vi "Set_TempHum_Calibration.vi"(2 "Path":path, 3 "Inside temp":dbl min=-7.0 max=7.0 step=0.01, 4 "Outside temp":dbl min=-7.0 max=7.0 step=0.01, 8 "Inside hum.":dbl, 9 "Outside hum":dbl) -> (0 "Cor. in temp":dbl, 1 "Cor. out temp":dbl, 5 "Cor. in hum":dbl, 6 "Cor. out hum":dbl, 7 "Calibration values set?":bool)   [LabVIEW 2012]
uses:
  <vilib>/Utility/config.llb/Write Key (Double).vi
  <vilib>/Utility/config.llb/Write Key (I32).vi
  VantagePro.dll
  <vilib>/Utility/config.llb/NI_LVConfig.lvlib
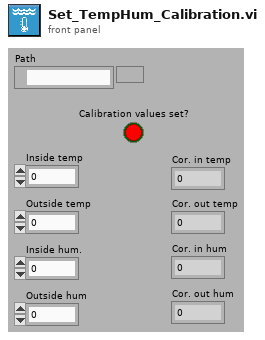
[diagram p1: front panel]
types:
  T1 = cluster{"In Temp":sgl, "Out Temp":sgl, "In Hum":u8, "Out Hum":u8, "Dum":i8, "Dum":i8, "Off In Temp":sgl, "Off Out Temp":sgl, "Off In Hum":i8, "Off Out Hum":i8}
  T2 = cluster{"In Temp":dbl, "Out Temp":dbl, "In Hum":dbl, "Out Hum":dbl}
  T3 = typedef "NI_LVConfig.lvlib/Config Data RefNum.ctl" = refnum<k1>
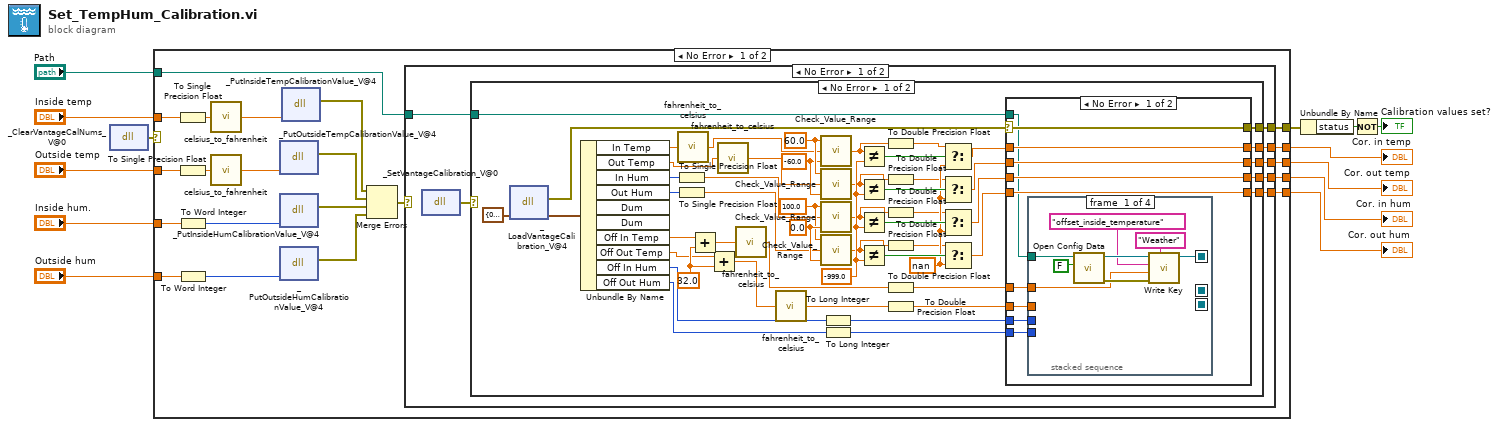
[diagram p0: block diagram]
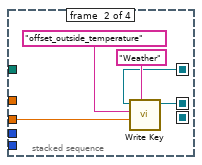
[diagram p2: hidden frame]
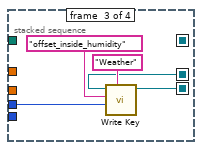
[diagram p3: hidden frame]
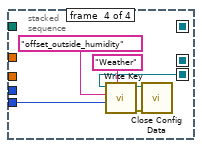
[diagram p4: hidden frame]
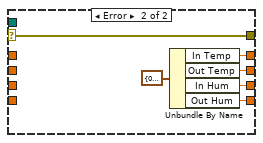
[diagram p5: hidden frame]
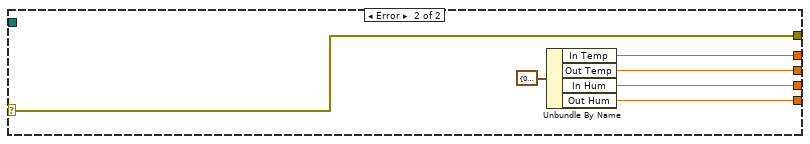
[diagram p6: hidden frame]
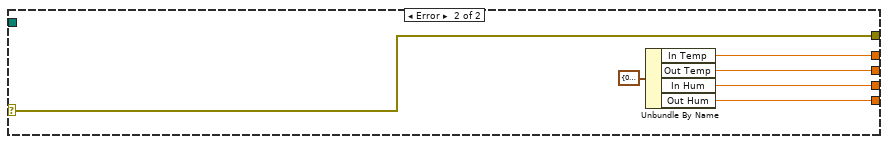
[diagram p7: hidden frame]
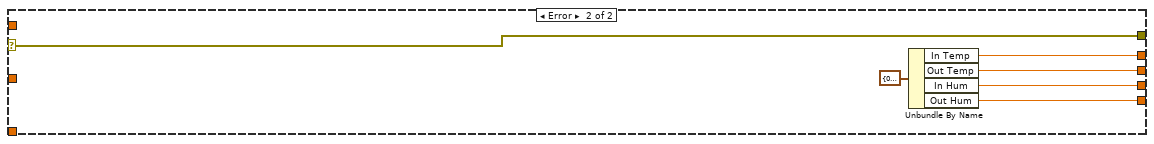
[diagram p8: hidden frame]
diagram:
  n1 = dll-call lib="C:/Users/Bob van Eijk/Desktop/LabView Projects 12/HiSPARC Weather Station/Develop/VantagePro.dll" fn="_ClearVantageCalNums_V@0" label="Clear Cal Nums"() -> (error out=w13:errorcluster)  [unwired: 4 in, 1 out]
  n2 = case shown="No Error" w13 {
    selector: w13 -> [_ w151]
    tunnel: "Inside temp" -> [w25 _]
    tunnel: "Inside hum." -> [w23 _]
    tunnel: "Outside temp" -> [w24 _]
    tunnel: "Outside hum" -> [w22 _]
    tunnel: "Path" -> [w31 _]
    tunnel: [w30 w151] -> w7
    tunnel: [w29 w149] -> w4
    tunnel: [w28 w148] -> w3
    tunnel: [w27 w147] -> w2
    tunnel: [w26 w146] -> w1
    frame No Error {
      n3 = To Single Precision Float(number=w25) -> (single precision float=w33:sgl)
      n4 = To Single Precision Float(number=w24) -> (single precision float=w34:sgl)
      n5 = To Word Integer(number=w23) -> (16bit integer=w15:i16)
      n6 = To Word Integer(number=w22) -> (16bit integer=w14:i16)
      n7 = call "celsius_to_fahrenheit.vi"("Celcius"=w33) -> ("Fahrenheit"=w21:sgl)
      n8 = call "celsius_to_fahrenheit.vi"("Celcius"=w34) -> ("Fahrenheit"=w16:sgl)
      n9 = dll-call lib="C:/Users/Bob van Eijk/Desktop/LabView Projects 12/HiSPARC Weather Station/Develop/VantagePro.dll" fn="_PutOutsideTempCalibrationValue_V@4" label="Put Out Temp Cal Val"("valValue"=w16) -> (error out=w19:errorcluster)  [unwired: 5 in, 1 out]
      n10 = dll-call lib="C:/Users/Bob van Eijk/Desktop/LabView Projects 12/HiSPARC Weather Station/Develop/VantagePro.dll" fn="_PutInsideHumCalibrationValue_V@4" label="Put In Hum Cal Val"("calValue"=w15) -> (error out=w18:errorcluster)  [unwired: 5 in, 1 out]
      n11 = dll-call lib="C:/Users/Bob van Eijk/Desktop/LabView Projects 12/HiSPARC Weather Station/Develop/VantagePro.dll" fn="_PutOutsideHumCalibrationValue_V@4" label="Put Out Hum Cal Val"("calValue"=w14) -> (error out=w17:errorcluster)  [unwired: 5 in, 1 out]
      n12 = dll-call lib="C:/Users/Bob van Eijk/Desktop/LabView Projects 12/HiSPARC Weather Station/Develop/VantagePro.dll" fn="_PutInsideTempCalibrationValue_V@4" label="Put In Temp Cal Val"("calValue"=w21) -> (error out=w20:errorcluster)  [unwired: 5 in, 1 out]
      n13 = Merge Errors(w20, w19, w18, w17) -> (w32:errorcluster)
      n14 = case shown="No Error" w32 {
        selector: w32 -> [_ w145]
        tunnel: [w39 w145] -> w30
        tunnel: w31 -> [w40 _]
        tunnel: [w38 w143] -> w29
        tunnel: [w37 w142] -> w28
        tunnel: [w36 w141] -> w27
        tunnel: [w35 w140] -> w26
        frame No Error {
          n15 = dll-call lib="C:/Users/Bob van Eijk/Desktop/LabView Projects 12/HiSPARC Weather Station/Develop/VantagePro.dll" fn="_SetVantageCalibration_V@0" label="Set cal. val."() -> (error out=w41:errorcluster)  [unwired: 4 in, 1 out]
          n16 = case shown="No Error" w41 {
            selector: w41 -> [_ w134]
            tunnel: [w77 w135] -> w35
            tunnel: [w78 w136] -> w36
            tunnel: [w79 w137] -> w37
            tunnel: [w80 w138] -> w38
            tunnel: [w75 w134] -> w39
            tunnel: w40 -> [w76 _]
            frame No Error {
              w55 = nan ("Data_input")
              w64 = sgl -999.0 ("Min")
              w74 = sgl 0.0 ("Min")
              w73 = sgl 100.0 ("Max")
              w71 = sgl -60.0 ("Min")
              w72 = sgl 60.0 ("Max")
              w90 = sgl 32.0
              n17 = dll-call lib="C:/Users/Bob van Eijk/Desktop/LabView Projects 12/HiSPARC Weather Station/Develop/VantagePro.dll" fn="_LoadVantageCalibration_V@4" label="Temp&hum data"("calibration"=T1 {"In Temp"=0.0, "Out Temp"=0.0, "In Hum"=0, "Out Hum"=0, "Dum"=0, "Dum"=0, "Off In Temp"=0.0, "Off Out Temp"=0.0, "Off In Hum"=0, "Off Out Hum"=0}) -> (error out=w42:errorcluster, "calibration"=w87:T1)  [unwired: 4 in, 1 out]
              n18 = Unbundle By Name(w87) -> ("In Temp"=w93:sgl, "Out Temp"=w85:sgl, "In Hum"=w68:u8, "Out Hum"=w67:u8, "Off In Temp"=w86:sgl, "Off Out Temp"=w89:sgl, "Off In Hum"=w82:i8, "Off Out Hum"=w81:i8)  [unwired: 2 out]
              n19 = To Single Precision Float(number=w68) -> (single precision float=w66:sgl)
              n20 = To Single Precision Float(number=w67) -> (single precision float=w65:sgl)
              n21 = call "fahrenheit_to_celsius.vi"("Fahrenheit"=w93) -> ("Celsius"=w70:sgl)
              n22 = Add(x=w86, y=w90) -> (x+y=w91:sgl)
              n23 = Add(x=w89, y=w90) -> (x+y=w92:sgl)
              n24 = call "fahrenheit_to_celsius.vi"("Fahrenheit"=w85) -> ("Celsius"=w69:sgl)
              n25 = call "fahrenheit_to_celsius.vi"("Fahrenheit"=w91) -> ("Celsius"=w84:sgl)
              n26 = call "fahrenheit_to_celsius.vi"("Fahrenheit"=w92) -> ("Celsius"=w83:sgl)
              n27 = call "Check_Value_Range.vi"("Min"=w71, "Data in"=w70, "Max"=w72) -> ("Data out"=w59:sgl)
              n28 = call "Check_Value_Range.vi"("Min"=w71, "Data in"=w69, "Max"=w72) -> ("Data out"=w58:sgl)
              n29 = call "Check_Value_Range.vi"("Min"=w74, "Data in"=w66, "Max"=w73) -> ("Data out"=w57:sgl)
              n30 = call "Check_Value_Range.vi"("Min"=w74, "Data in"=w65, "Max"=w73) -> ("Data out"=w56:sgl)
              n31 = To Long Integer(number=w82) -> (32bit integer=w50:i32)
              n32 = To Long Integer(number=w81) -> (32bit integer=w49:i32)
              n33 = Not Equal?(x=w59, y=w64) -> (x != y?=w63:bool)
              n34 = Not Equal?(x=w58, y=w64) -> (x != y?=w61:bool)
              n35 = Not Equal?(x=w57, y=w64) -> (x != y?=w60:bool)
              n36 = Not Equal?(x=w56, y=w64) -> (x != y?=w62:bool)
              n37 = To Double Precision Float(number=w59) -> (double precision float=w46:dbl)
              n38 = To Double Precision Float(number=w58) -> (double precision float=w45:dbl)
              n39 = To Double Precision Float(number=w57) -> (double precision float=w44:dbl)
              n40 = To Double Precision Float(number=w56) -> (double precision float=w43:dbl)
              n41 = To Double Precision Float(number=w84) -> (double precision float=w48:dbl)
              n42 = To Double Precision Float(number=w83) -> (double precision float=w47:dbl)
              n43 = Select(t=w46, s=w63, f=w55) -> (s? t:f=w54:dbl)
              n44 = Select(t=w45, s=w61, f=w55) -> (s? t:f=w53:dbl)
              n45 = Select(t=w44, s=w60, f=w55) -> (s? t:f=w52:dbl)
              n46 = Select(t=w43, s=w62, f=w55) -> (s? t:f=w51:dbl)
              n47 = case shown="No Error" w42 {
                selector: w42 -> [w103 w133]
                tunnel: w54 -> [w102 _]
                tunnel: w53 -> [w101 _]
                tunnel: w52 -> [w100 _]
                tunnel: w51 -> [w99 _]
                tunnel: w48 -> [w94 _]
                tunnel: w47 -> [w95 _]
                tunnel: w50 -> [w96 _]
                tunnel: w49 -> [w97 _]
                tunnel: [w102 w131] -> w80
                tunnel: [w101 w130] -> w79
                tunnel: [w100 w129] -> w78
                tunnel: [w99 w128] -> w77
                tunnel: w76 -> [w98 _]
                tunnel: [w103 w133] -> w75
                frame No Error {
                  n48 = stacked-sequence {
                    seq-local: [w108 _ _ _] -> [_ w114 _ _]
                    seq-local: [_ _ w118 _] -> [_ _ _ w122]
                    seq-local: [_ w112 _ _] -> [_ _ w117 _]
                    tunnel: w98 -> [w109 _ _ _]
                    tunnel: w94 -> [w104 _ _ _]
                    tunnel: w96 -> [_ _ w119 _]
                    tunnel: w95 -> [_ w113 _ _]
                    tunnel: w97 -> [_ _ _ w123]
                    frame #0 {
                      n49 = call <vilib>:"Open Config Data.vi"("create file if necessary (T)"=FALSE, "configuration file path"=w109) -> ("error out"=w106:errorcluster, "refnum"=w110:T3)  [unwired: 7 in, 1 out]
                      n50 = call-poly <vilib>:"Write Key.vi"("section"="Weather" ("key"), "error in (no error)"=w106, "value"=w104, "key"="offset_inside_temperature", "refnum"=w110) -> ("refnum out"=w108:T3)  [unwired: 4 in, 2 out]
                    }
                    frame #1 {
                      n51 = call-poly <vilib>:"Write Key.vi"("section"="Weather" ("key"), "value"=w113, "key"="offset_outside_temperature", "refnum"=w114) -> ("refnum out"=w112:T3)  [unwired: 5 in, 2 out]
                    }
                    frame #2 {
                      n52 = call-poly <vilib>:"Write Key.vi"("section"="Weather" ("key"), "value"=w119, "key"="offset_inside_humidity", "refnum"=w117) -> ("refnum out"=w118:T3)  [unwired: 5 in, 2 out]
                    }
                    frame #3 {
                      n53 = call-poly <vilib>:"Write Key.vi"("section"="Weather" ("key"), "value"=w123, "key"="offset_outside_humidity", "refnum"=w122) -> ("error out"=w124:errorcluster, "refnum out"=w125:T3)  [unwired: 5 in, 1 out]
                      n54 = call <vilib>:"Close Config Data.vi"("error in (no error)"=w124, "refnum"=w125) -> ()  [unwired: 8 in, 2 out]
                    }
                  }
                }
                frame Error {
                  n55 = Unbundle By Name(T2 {"In Temp"=0.0, "Out Temp"=0.0, "In Hum"=0.0, "Out Hum"=0.0}) -> ("In Temp"=w131:dbl, "Out Temp"=w130:dbl, "In Hum"=w129:dbl, "Out Hum"=w128:dbl)
                }
              }
            }
            frame Error {
              n56 = Unbundle By Name(T2 {"In Temp"=0.0, "Out Temp"=0.0, "In Hum"=0.0, "Out Hum"=0.0}) -> ("In Temp"=w138:dbl, "Out Temp"=w137:dbl, "In Hum"=w136:dbl, "Out Hum"=w135:dbl)
            }
          }
        }
        frame Error {
          n57 = Unbundle By Name(T2 {"In Temp"=0.0, "Out Temp"=0.0, "In Hum"=0.0, "Out Hum"=0.0}) -> ("In Temp"=w143:dbl, "Out Temp"=w142:dbl, "In Hum"=w141:dbl, "Out Hum"=w140:dbl)
        }
      }
    }
    frame Error {
      n58 = Unbundle By Name(T2 {"In Temp"=0.0, "Out Temp"=0.0, "In Hum"=0.0, "Out Hum"=0.0}) -> ("In Temp"=w149:dbl, "Out Temp"=w148:dbl, "In Hum"=w147:dbl, "Out Hum"=w146:dbl)
    }
  }
  "Cor. in temp" <- w4
  "Cor. out temp" <- w3
  "Cor. in hum" <- w2
  "Cor. out hum" <- w1
  n59 = Unbundle By Name(w7) -> ("status"=w6:bool)
  n60 = Not(x=w6) -> (.not. x?=→"Calibration values set?":bool)
